vi "Create schedule.vi"(8 "Action":T1 items=["Turn off all", "Turn on all", "Fan on", "Fan off", "Light on", "Light off"], 9 "Repeat":T2, 11 "Time in":timestamp) -> (0 "arr out":string[](array[string]))   [LabVIEW 2018]
uses:
  Global variable.vi
  5000a914-0bc1-46bc-b5eb-f63c1aee4f0b.vi
  Typedef/Repeat.ctl
  Typedef/Action.ctl
  Typedef/Schedule.ctl
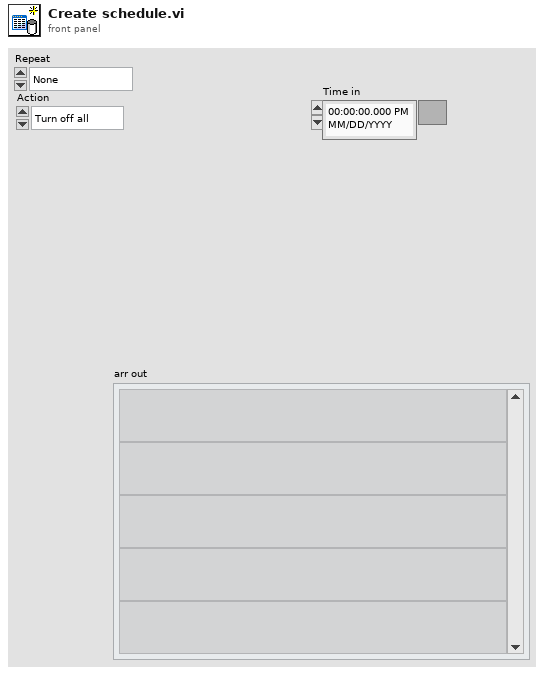
[diagram p1: front panel]
types:
  T1 = typedef "Action.ctl" = u16
  T2 = typedef "Repeat.ctl" = enum16{"None", "Every hour", "Every day", "Every week", "Every month"}
  T3 = typedef "Schedule.ctl" = cluster{"Start time":timestamp, "Repeat":T2, "Action":T1}
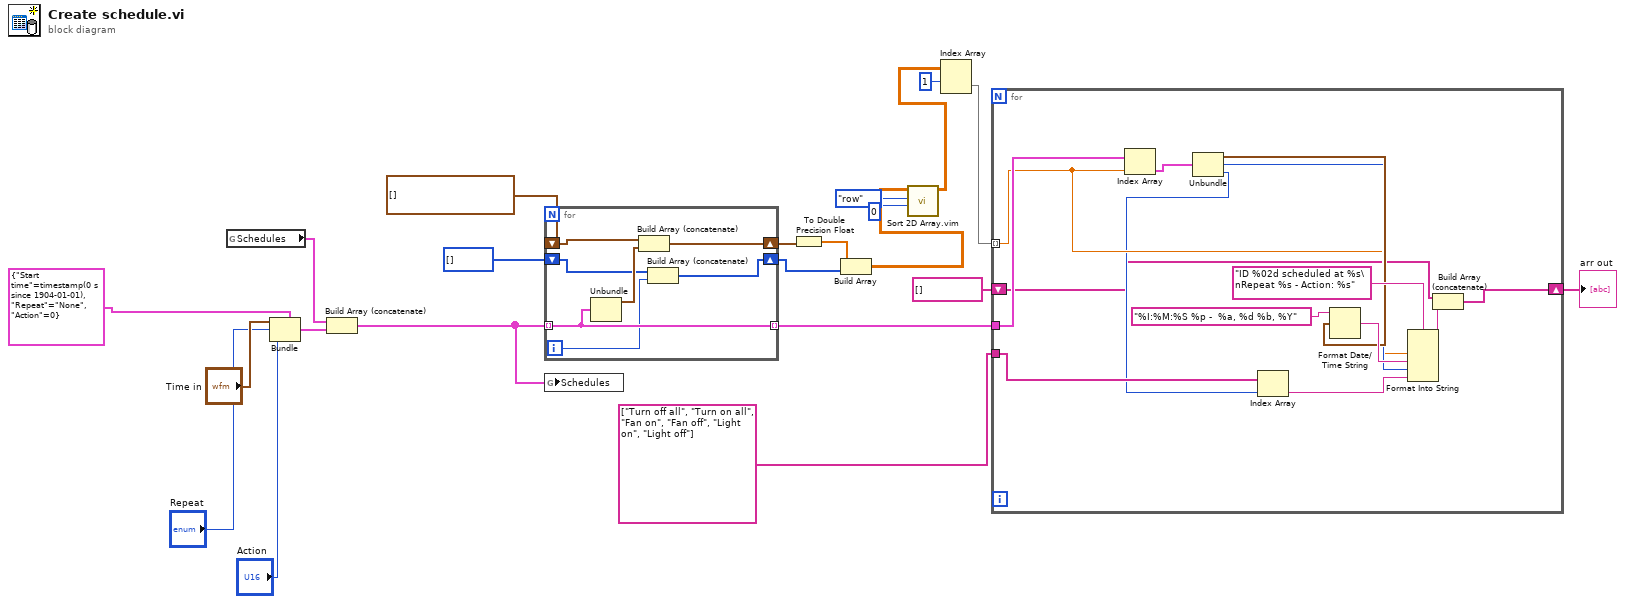
[diagram p0: block diagram]
diagram:
  n1 = global read "Global variable.vi" "Schedules"() -> (w21:T3[])
  n2 = Bundle(cluster=T3 {"Start time"=timestamp(0 s since 1904-01-01), "Repeat"=enum."None", "Action"=0} ("Cluster"), "Start time"="Time in", "Repeat"="Repeat", "Action"="Action") -> (w20:T3)
  n3 = Build Array (concatenate)(w21, w20) -> (w19:T3[])
  n4 = for {
    tunnel: w19 -> [w28] mode=indexing
    shift-right: [w26] -> w12
    shift-left: timestamp[] [] -> [w24]
    tunnel: [w28] -> w18 mode=indexing
    shift-right: [w25] -> w13
    shift-left: i32[] [] -> [w23]
    i -> [w27]
    n5 = Unbundle(w28) -> ("Start time"=w29:timestamp)  [unwired: 2 out]
    n6 = Build Array (concatenate)(w24, w29) -> (w26:timestamp[])
    n7 = Build Array (concatenate)(w23, w27) -> (w25:i32[])
  }
  n8 = global write "Global variable.vi" "Schedules"(w19) -> ()
  n9 = To Double Precision Float(number=w12) -> (double precision float=w11:dbl[])
  n10 = Build Array(w11, w13) -> (w10:dbl[][])
  n11 = call "Sort 2D Array.vim"("index"=0, "dimension to index (column)"=enum16{"column", "row"}."row", "2D array"=w10) -> ("sorted 2D array"=w7:dbl[][])  [unwired: 7 in, 1 out]
  n12 = Index Array(array=w7, index (row)=1) -> (element=w5:dbl[])  [unwired: 1 in]
  n13 = for {
    tunnel: w18 -> [w43]
    shift-right: [w37] -> w17
    shift-left: string[] [] -> [w30]
    tunnel: string[] ["Turn off all", "Turn on all", "Fan on", "Fan off", "Light on", "Light off"] -> [w33]
    tunnel: w5 -> [w34] mode=indexing
    n14 = Index Array(array=w43, index=w34) -> (element=w42:T3)
    n15 = Unbundle(w42) -> ("Start time"=w36:timestamp, "Repeat"=w35:T2, "Action"=w32:T1)
    n16 = Index Array(array=w33, index=w32) -> (element=w31:string)
    n17 = Format Date/Time String(time format string (%c)="%I:%M:%S %p -  %a, %d %b, %Y", seconds (now)=w36) -> (date/time string=w40:string)  [unwired: 1 in]
    n18 = Format Into String(format string="ID %02d scheduled at %s\nRepeat %s - Action: %s" ("FMT string"), w34, w40, w35, w31) -> (resulting string=w41:string)  [unwired: 2 in, 1 out]
    n19 = Build Array (concatenate)(w30, w41) -> (w37:string[])
  }
  "arr out" <- w17
